vi "disconnect.vi"(8 "error in":errorcluster, 11 "MQTT client in":refnum<class "MQTT client.lvclass">) -> (0 "error out":errorcluster, 3 "MQTT client out":refnum<class "MQTT client.lvclass">)   [LabVIEW 2014, in "MQTT client.lvclass"]
uses:
  MQTT client.lvclass
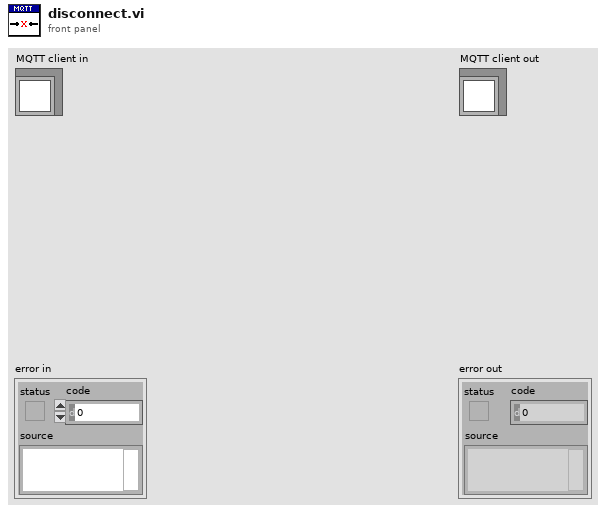
[diagram p1: front panel]
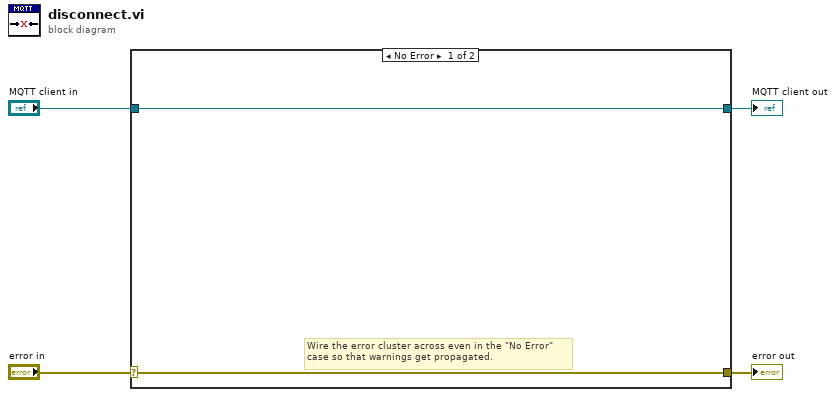
[diagram p0: block diagram]
diagram:
  n1 = case shown="No Error" "error in" {
    selector: "error in" -> [w5 w8]
    tunnel: [w5 w8] -> w3
    tunnel: [w6 w7] -> w1
    tunnel: "MQTT client in" -> [w6 w7]
    frame No Error {
      # "Wire the error cluster across even in the \"No Error\"\ncase so that warnings get propagated."
    }
    frame Error {
    }
  }
  "error out" <- w3
  "MQTT client out" <- w1
